vi "Avocent_controller.vi"() -> ()   [LabVIEW 2013]
doc: "Example of using standard HTTP protocol for recieving a web site (the HTML source)\n\n\nThis example uses the GET command. For general information about the HTTP protocol and other commands go to\nhttp://www.w3.org/Protocols\n\n\nBjornar Svingen\nbjornar.svingen@sintef.no bjornar.svingen@ktv.no"
uses:
  <vilib>/Utility/config.llb/Read Key (String).vi
  <vilib>/Utility/config.llb/NI_LVConfig.lvlib
panel:
  in  "Set to all on/off av2":bool
  in  "Set to all on/off av1":bool
  in  "toggle av2":bool
  in  "toggle av1":bool
  out "Avocent Labels Av2":string[](array[string])
  out "Avocent Labels Av1":string[](array[string])
  in  "Set to current values 2":bool
  in  "Set to current values":bool
  in  "Get status 2":bool
  in  "send command 2":bool
  out "Power indicator 2":bool[](array[boolean])=[FALSE, FALSE, FALSE, FALSE, FALSE, FALSE, FALSE, FALSE, FALSE, FALSE, FALSE, FALSE, FALSE, TRUE, TRUE, TRUE, FALSE, FALSE, FALSE, FALSE, FALSE, FALSE, FALSE, FALSE, FALSE, FALSE, FALSE, FALSE, FALSE, FALSE, FALSE, FALSE] caption="Power indicator"
  in  "Set switches 2":bool[](array[boolean])=[FALSE, FALSE, FALSE, FALSE, FALSE, FALSE, FALSE, FALSE, FALSE, FALSE, FALSE, FALSE, FALSE, TRUE, TRUE, TRUE] caption="Set Switches"
  in  "Avocent 2 IP":string="192.168.15.5"
  in  "Set switches":bool[](array[boolean])=[FALSE, TRUE, TRUE, FALSE, TRUE, TRUE, TRUE, TRUE, TRUE, TRUE, TRUE, FALSE, TRUE, TRUE, TRUE, FALSE] caption="Set Switches"
  out "Power indicator":bool[](array[boolean])=[FALSE, TRUE, TRUE, FALSE, TRUE, TRUE, TRUE, TRUE, TRUE, TRUE, TRUE, FALSE, TRUE, TRUE, TRUE, FALSE, FALSE, FALSE, FALSE, FALSE, FALSE, FALSE, FALSE, FALSE, FALSE, FALSE, FALSE, FALSE, FALSE, FALSE, FALSE, FALSE]
  in  "Get status":bool
  in  "send command":bool
  in  "Exit":bool
  in  "Avocent 1 IP":string="192.168.14.88"
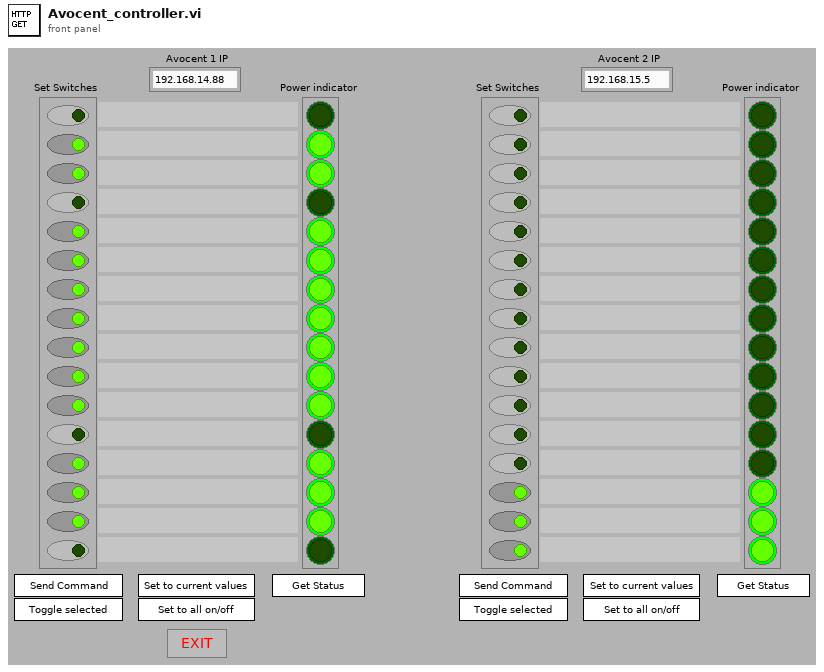
[diagram p1: front panel]
types:
  T1 = enum32{"invalid app kind", "Development System", "Run Time System", "Student Edition", "Embedded LabVIEW", "Evaluation", "Custom"}
  T2 = enum32{"Invalid", "Standard", "Closed", "Hidden", "Minimized", "Maximized"}
  T3 = cluster{"Core":cluster{"Current VI Reference":refnum<vi>, "Close Panel on Exit?":bool}, "HTTP Command":string, "Set Switch Status":bool[], "Power Status":string, "Toggle On/Off":bool, "Set all On/Off":bool}
  T4 = cluster{"Current VI Reference":refnum<vi>, "Close Panel on Exit?":bool}
  T5 = typedef "NI_LVConfig.lvlib/Config Data RefNum.ctl" = refnum<k1>
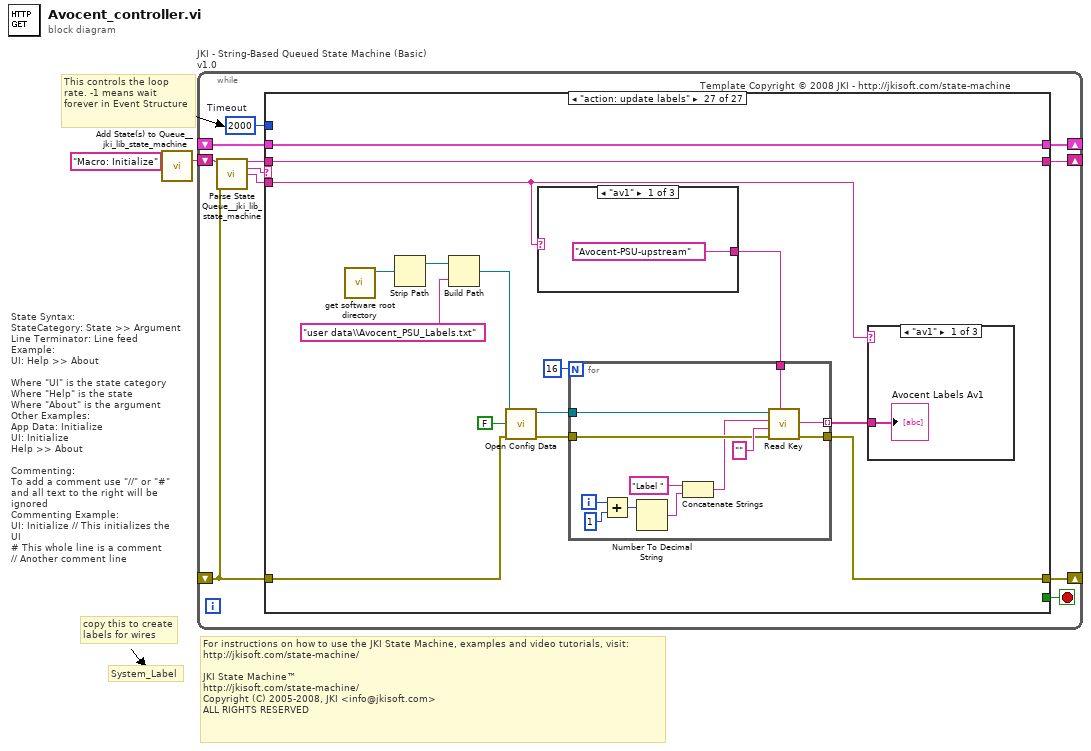
[diagram p0: block diagram]
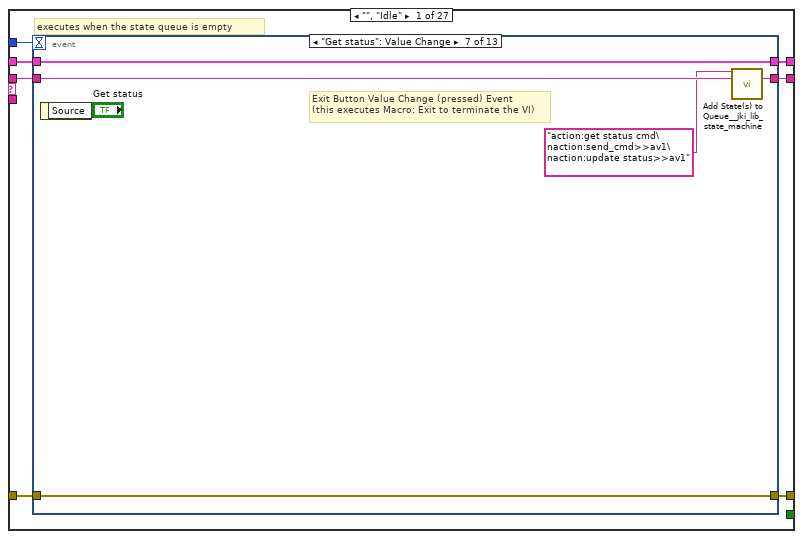
[diagram p2: hidden frame]
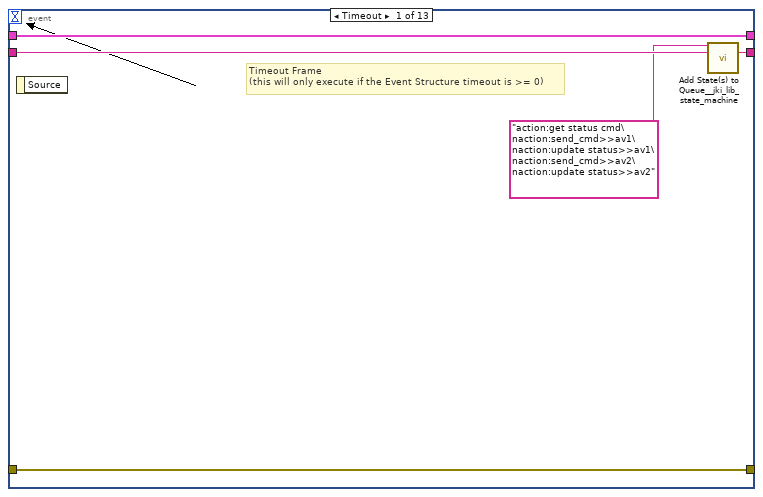
[diagram p3: hidden frame]
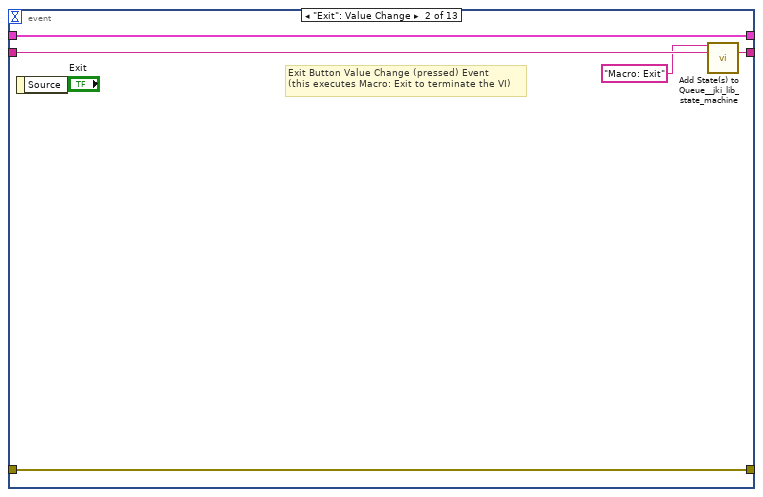
[diagram p4: hidden frame]
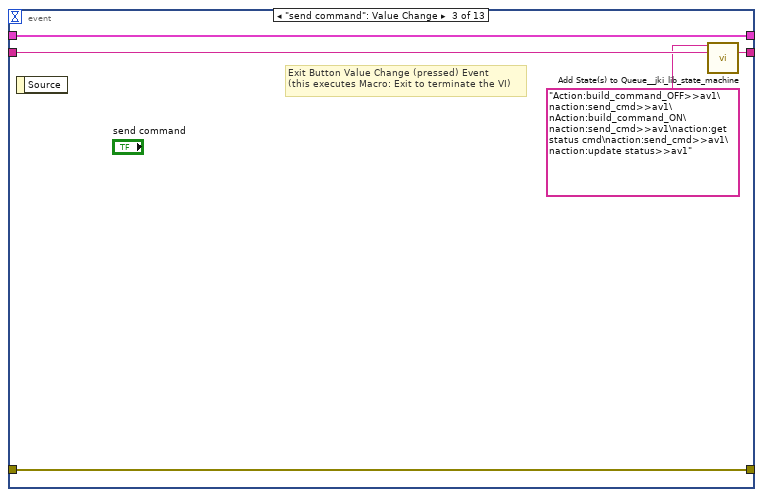
[diagram p5: hidden frame]
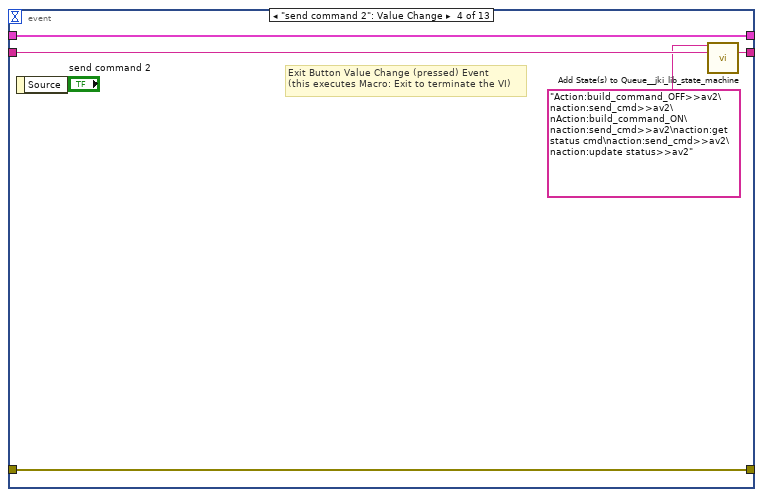
[diagram p6: hidden frame]
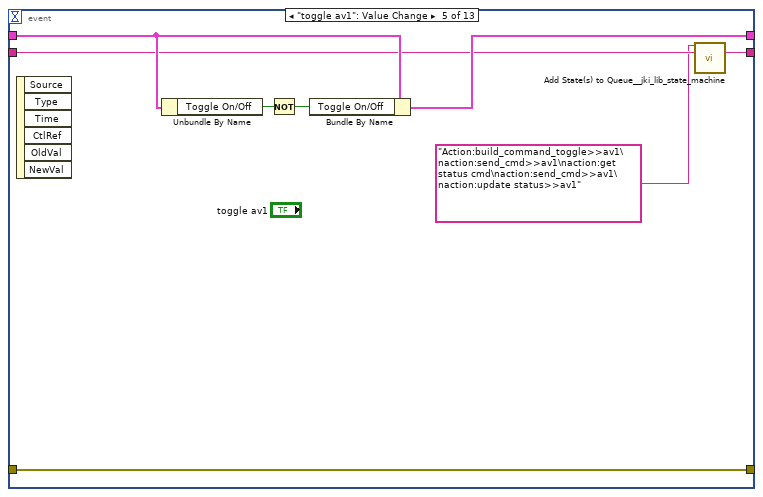
[diagram p7: hidden frame]
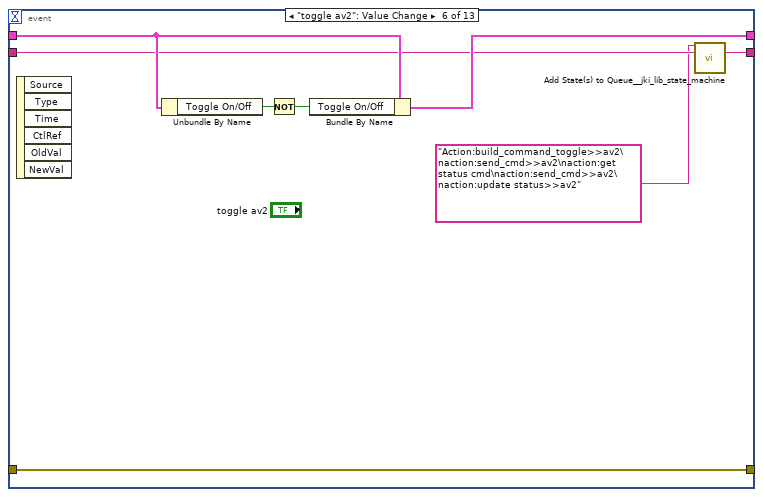
[diagram p8: hidden frame]
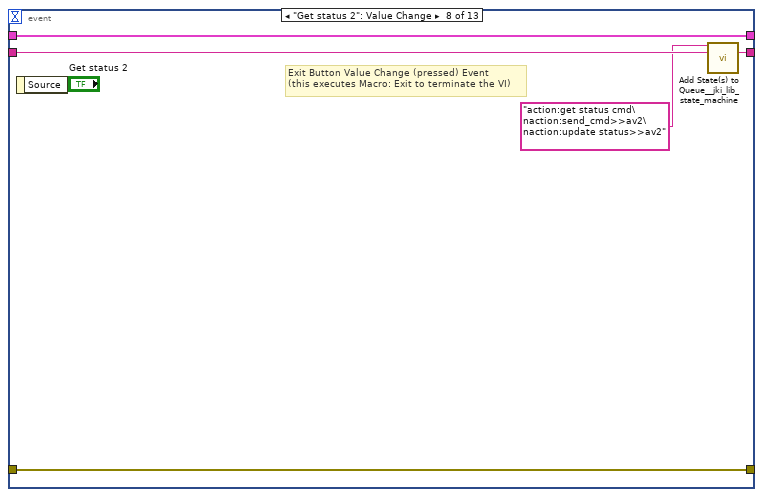
[diagram p9: hidden frame]
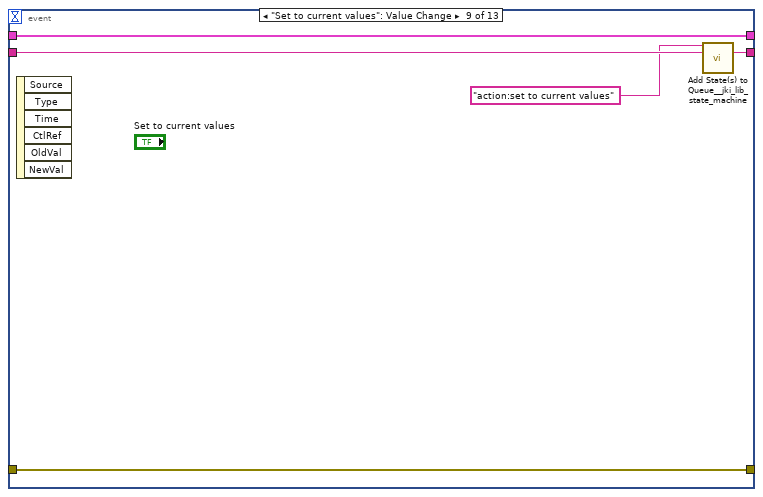
[diagram p10: hidden frame]
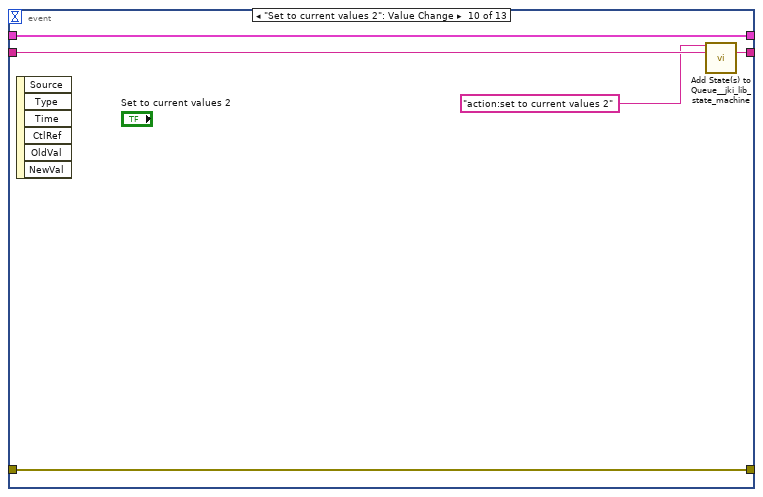
[diagram p11: hidden frame]
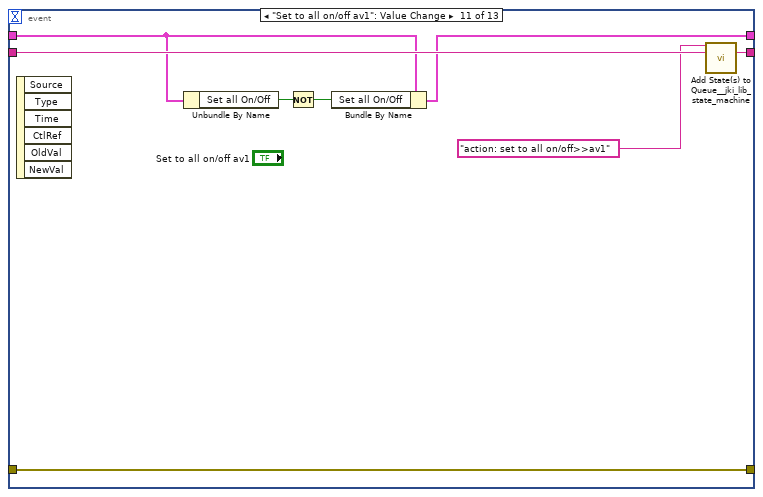
[diagram p12: hidden frame]
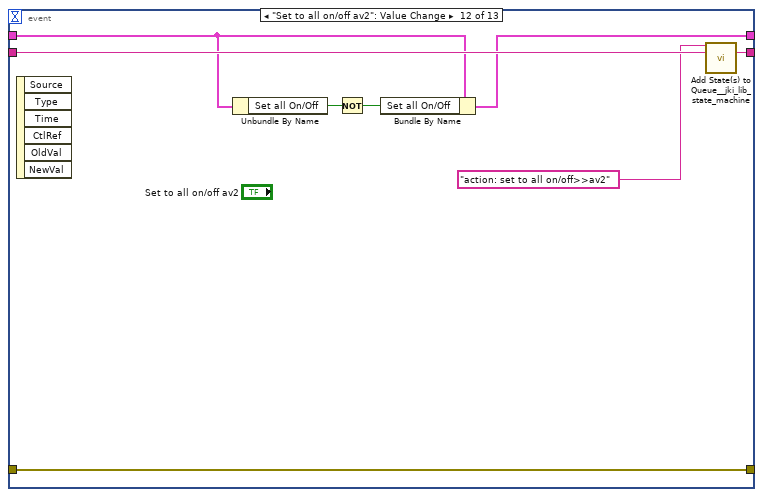
[diagram p13: hidden frame]
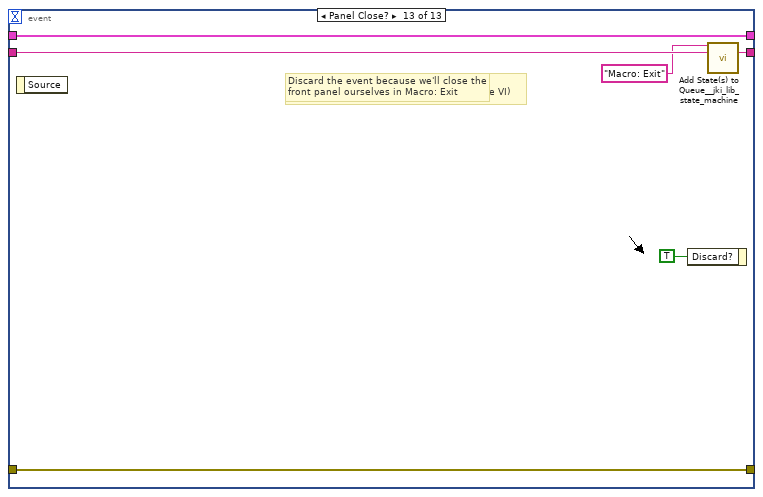
[diagram p14: hidden frame]
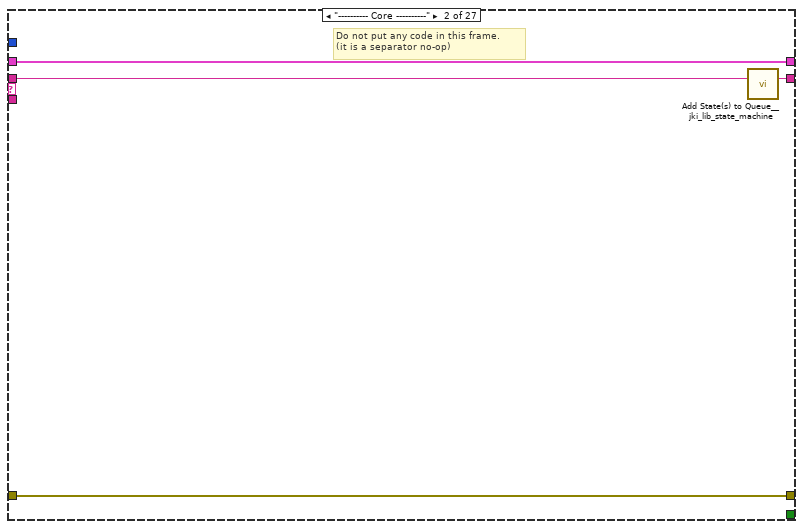
[diagram p15: hidden frame]
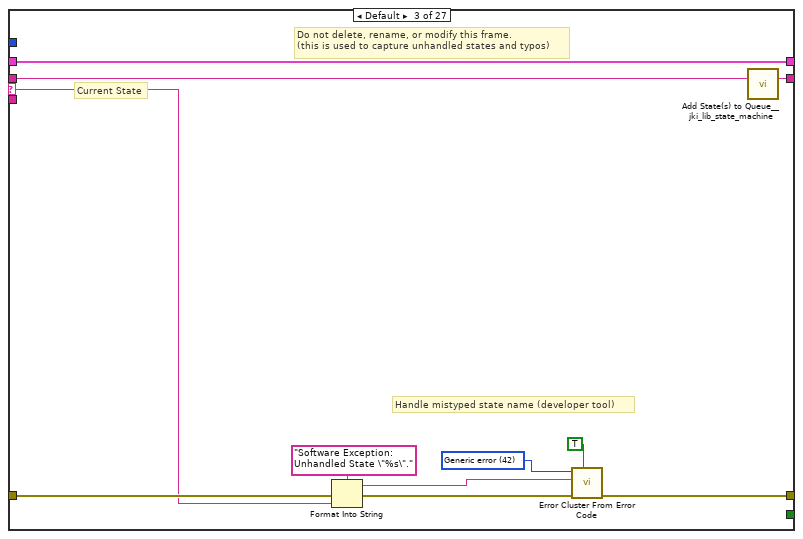
[diagram p16: hidden frame]
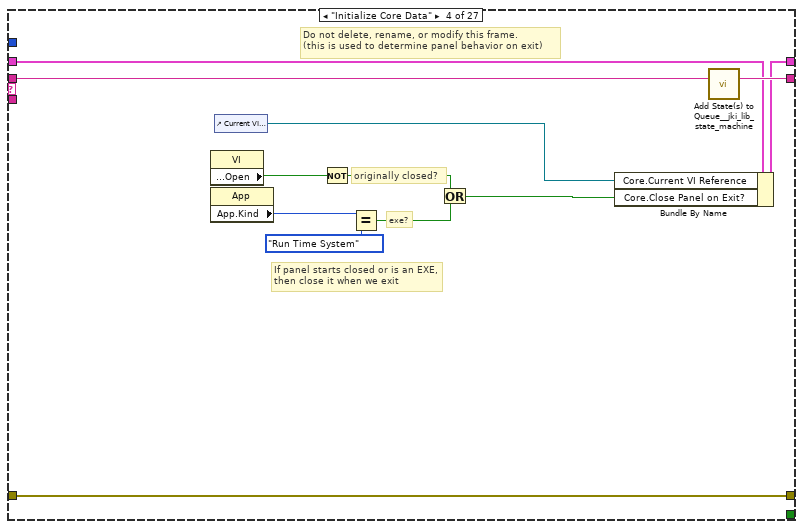
[diagram p17: hidden frame]
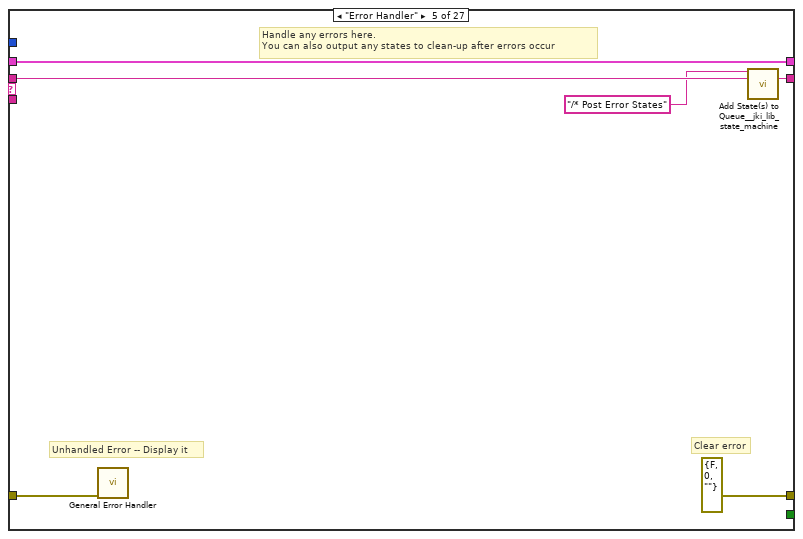
[diagram p18: hidden frame]
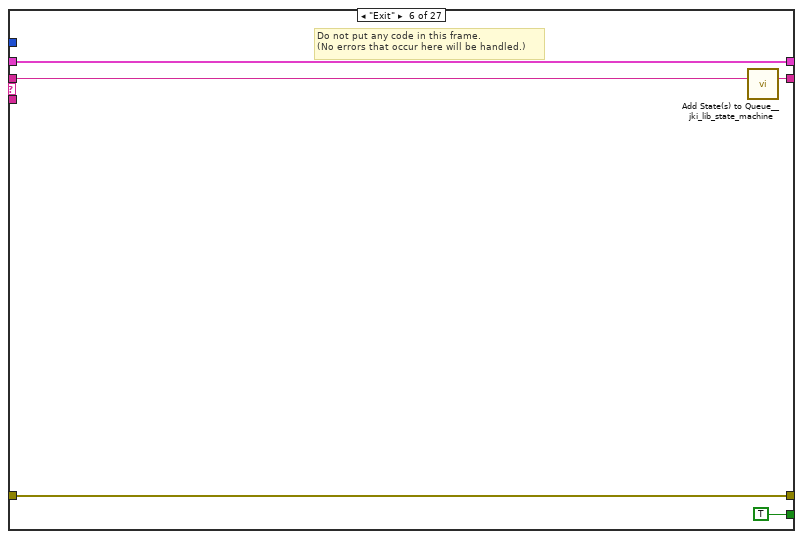
[diagram p19: hidden frame]
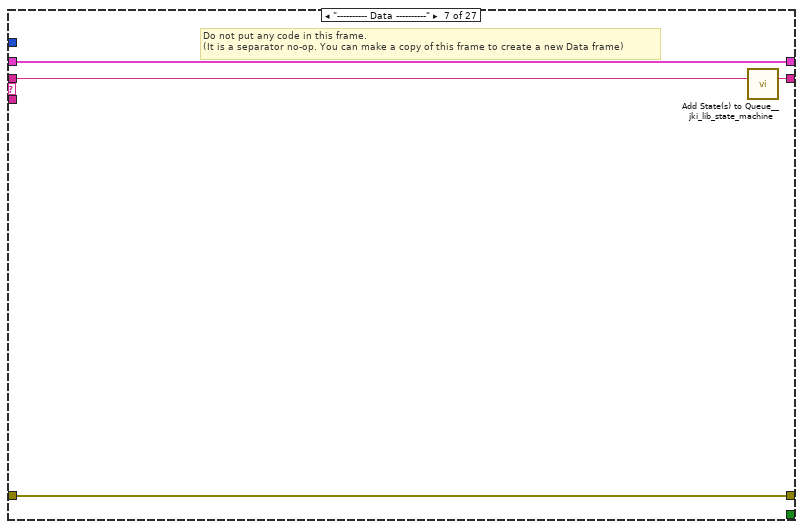
[diagram p20: hidden frame]
diagram:
  # "For instructions on how to use the JKI State Machine, examples and video tutorials, visit:\nhttp://jkisoft.com/state-machine/\n\nJKI State Machine™\nhttp://jkisoft.com/state-machine/\nCopyright (C) 2005-2008, JKI <info@jkisoft.com>\nALL RIGHTS RESERVED"
  # "State Syntax:\nStateCategory: State >> Argument\nLine Terminator: Line feed\nExample:\nUI: Help >> About\n\nWhere \"UI\" is the state category\nWhere \"Help\" is the state\nWhere \"About\" is the argument\nOther Examples:\nApp Data: Initialize\nUI: Initialize\nHelp >> About\n\nCommenting:\nTo add a comment use \"//\" or \"#\" and all text to the right will be ignored\nCommenting Example:\nUI: Initialize // This initializes the UI\n# This whole line is a comment\n// Another comment line"
  # "copy this to create labels for wires"
  # "This controls the loop rate. -1 means wait forever in Event Structure"
  # "System_Label"
  n1 = call <vilib>:"Add State(s) to Queue__jki_lib_state_machine.vi"("State(s) in (\"\")"="Macro: Initialize") -> ("States Out"=w2:string)  [unwired: 14 in]
  n2 = while "JKI - String-Based Queued State Machine (Basic) v1.0" {
    shift-right: [w6] -> _
    shift-left: _ -> [w5]
    shift-right: [w9] -> _
    shift-left: _ -> [w3]
    shift-right: [w8] -> _
    shift-left: w2 -> [w10]
    stop <- w7 stop-if-true
    w4 = 2000  # Timeout
    # "Template Copyright © 2008 JKI - http://jkisoft.com/state-machine"
    n3 = call <vilib>:"Parse State Queue__jki_lib_state_machine.vi"("State Queue"=w10, "Error In (no error)"=w3) -> ("Remaining States"=w12:string, "Current State"=w13:string, "Arguments"=w11:string)  [unwired: 11 in]
    n4 = case shown="\"action: update labels\"" w13 {
      selector: w13 -> [_ _ w103 _ _ _ _ _ _ _ _ _ _ _ _ _ _ _ _ _ _ _ _ _ _ _ _]
      tunnel: w12 -> [w20 w102 w107 w125 w131 w136 w140 w150 w156 w160 w164 w170 w181 w207 w212 w222 w226 w228 w252 w272 w277 w297 w316 w323 w330 w336 w364]
      tunnel: w11 -> [_ _ _ _ _ _ _ _ _ _ _ w165 w175 _ _ _ _ w231 w253 _ w279 w300 _ _ _ w337 w351]
      tunnel: w5 -> [w18 w99 w105 w116 w128 w134 w137 _ w151 w157 w162 w168 w177 w204 w209 w219 w223 w233 w256 w268 w278 w301 w313 w321 w328 w332 w365]
      tunnel: [w17 w100 w109 w122 errorcluster {"status"=FALSE, "code"=0, "source"=""} ("error out") w133 w138 w147 w152 w158 w161 w166 w178 w205 w210 w220 w224 w236 w250 w270 w280 w298 w314 w318 w326 w338 w355] -> w9
      tunnel: w3 -> [w16 w100 w108 w122 w127 w133 w138 w147 w153 w158 w161 w167 w179 w205 w210 w220 w224 w230 w251 w270 w281 w299 w314 w319 w327 w339 w356]
      tunnel: [w19 w101 w106 w124 w130 w135 w139 w149 w155 w159 w163 w169 w180 w206 w211 w221 w225 w238 w257 w271 w283 w302 w315 w322 w329 w340 w364] -> w8
      tunnel: [_ _ _ _ _ TRUE _ _ _ _ _ _ _ _ _ _ _ _ _ _ _ _ _ _ _ _ _] -> w7
      tunnel: [w15 w99 w105 w123 w128 w134 w137 w148 w151 w157 w162 w168 w177 w204 w209 w219 w223 w232 w254 w269 w282 w301 w312 w321 w328 w332 w365] -> w6
      tunnel: w4 -> [w14 _ _ _ _ _ _ _ _ _ _ _ _ _ _ _ _ _ _ _ _ _ _ _ _ _ _]
      frame "", "Idle" {
        # "executes when the state queue is empty"
        n5 = event shown="[6] \"Get status\": Value Change" {
          selector: _ -> [_ _ _ _ _ _ _ _ _ _ _ _ _]
          dyn-events: _ -> [_ _ _ _ _ _ _ _ _ _ _ _ _]
          timeout: w14 -> [_ _ _ _ _ _ _ _ _ _ _ _ _]
          tunnel: w20 -> [w25 w30 w35 w40 w43 w51 w61 w66 w68 w73 w82 w90 w98]
          tunnel: [w24 w29 w34 w39 w42 w50 w60 w65 w69 w74 w83 w91 w97] -> w19
          tunnel: w18 -> [w22 w27 w32 w37 w46 w54 w58 w63 w71 w76 w78 w86 w95]
          tunnel: [w23 w28 w33 w38 w48 w56 w59 w64 w70 w75 w84 w92 w96] -> w17
          tunnel: w16 -> [w23 w28 w33 w38 w48 w56 w59 w64 w70 w75 w84 w92 w96]
          tunnel: [w22 w27 w32 w37 w47 w55 w58 w63 w71 w76 w77 w85 w95] -> w15
          event Timeout {
            # "Timeout Frame\n(this will only execute if the Event Structure timeout is >= 0)"
            n6 = event-data() -> ()  [unwired: 1 in, 1 out]
            n7 = call <vilib>:"Add State(s) to Queue__jki_lib_state_machine.vi"("State(s) in Front (\"\")"="action:get status cmd\naction:send_cmd>>av1\naction:update status>>av1\naction:send_cmd>>av2\naction:update status>>av2", "State(s) in (\"\")"=w25) -> ("States Out"=w24:string)  [unwired: 13 in]
          }
          event "Exit": Value Change {
            # "Exit Button Value Change (pressed) Event\n(this executes Macro: Exit to terminate the VI)"
            n8 = event-data() -> ()  [unwired: 1 in, 1 out]
            n9 = call <vilib>:"Add State(s) to Queue__jki_lib_state_machine.vi"("State(s) in Front (\"\")"="Macro: Exit", "State(s) in (\"\")"=w30) -> ("States Out"=w29:string)  [unwired: 13 in]
          }
          event "send command": Value Change {
            # "Exit Button Value Change (pressed) Event\n(this executes Macro: Exit to terminate the VI)"
            n10 = event-data() -> ()  [unwired: 1 in, 1 out]
            n11 = call <vilib>:"Add State(s) to Queue__jki_lib_state_machine.vi"("State(s) in Front (\"\")"="Action:build_command_OFF>>av1\naction:send_cmd>>av1\nAction:build_command_ON\naction:send_cmd>>av1\naction:get status cmd\naction:send_cmd>>av1\naction:update status>>av1", "State(s) in (\"\")"=w35) -> ("States Out"=w34:string)  [unwired: 13 in]
          }
          event "send command 2": Value Change {
            # "Exit Button Value Change (pressed) Event\n(this executes Macro: Exit to terminate the VI)"
            n12 = event-data() -> ()  [unwired: 1 in, 1 out]
            n13 = call <vilib>:"Add State(s) to Queue__jki_lib_state_machine.vi"("State(s) in Front (\"\")"="Action:build_command_OFF>>av2\naction:send_cmd>>av2\nAction:build_command_ON\naction:send_cmd>>av2\naction:get status cmd\naction:send_cmd>>av2\naction:update status>>av2", "State(s) in (\"\")"=w40) -> ("States Out"=w39:string)  [unwired: 13 in]
          }
          event "toggle av1": Value Change {
            n14 = event-data() -> ()  [unwired: 1 in, 6 out]
            n15 = Unbundle By Name(w46) -> ("Toggle On/Off"=w45:bool)
            n16 = Not(x=w45) -> (.not. x?=w44:bool)
            n17 = Bundle By Name(cluster=w46, "Toggle On/Off"=w44) -> (w47:T3)
            n18 = call <vilib>:"Add State(s) to Queue__jki_lib_state_machine.vi"("State(s) in Front (\"\")"="Action:build_command_toggle>>av1\naction:send_cmd>>av1\naction:get status cmd\naction:send_cmd>>av1\naction:update status>>av1", "State(s) in (\"\")"=w43) -> ("States Out"=w42:string)  [unwired: 13 in]
          }
          event "toggle av2": Value Change {
            n19 = event-data() -> ()  [unwired: 1 in, 6 out]
            n20 = Unbundle By Name(w54) -> ("Toggle On/Off"=w53:bool)
            n21 = Not(x=w53) -> (.not. x?=w52:bool)
            n22 = Bundle By Name(cluster=w54, "Toggle On/Off"=w52) -> (w55:T3)
            n23 = call <vilib>:"Add State(s) to Queue__jki_lib_state_machine.vi"("State(s) in Front (\"\")"="Action:build_command_toggle>>av2\naction:send_cmd>>av2\naction:get status cmd\naction:send_cmd>>av2\naction:update status>>av2", "State(s) in (\"\")"=w51) -> ("States Out"=w50:string)  [unwired: 13 in]
          }
          event "Get status": Value Change {
            # "Exit Button Value Change (pressed) Event\n(this executes Macro: Exit to terminate the VI)"
            n24 = event-data() -> ()  [unwired: 1 in, 1 out]
            n25 = call <vilib>:"Add State(s) to Queue__jki_lib_state_machine.vi"("State(s) in Front (\"\")"="action:get status cmd\naction:send_cmd>>av1\naction:update status>>av1", "State(s) in (\"\")"=w61) -> ("States Out"=w60:string)  [unwired: 13 in]
          }
          event "Get status 2": Value Change {
            # "Exit Button Value Change (pressed) Event\n(this executes Macro: Exit to terminate the VI)"
            n26 = event-data() -> ()  [unwired: 1 in, 1 out]
            n27 = call <vilib>:"Add State(s) to Queue__jki_lib_state_machine.vi"("State(s) in Front (\"\")"="action:get status cmd\naction:send_cmd>>av2\naction:update status>>av2", "State(s) in (\"\")"=w66) -> ("States Out"=w65:string)  [unwired: 13 in]
          }
          event "Set to current values": Value Change {
            n28 = event-data() -> ()  [unwired: 1 in, 6 out]
            n29 = call <vilib>:"Add State(s) to Queue__jki_lib_state_machine.vi"("State(s) in Front (\"\")"="action:set to current values" ("State(s) in Front (\"\")"), "State(s) in (\"\")"=w68) -> ("States Out"=w69:string)  [unwired: 13 in]
          }
          event "Set to current values 2": Value Change {
            n30 = event-data() -> ()  [unwired: 1 in, 6 out]
            n31 = call <vilib>:"Add State(s) to Queue__jki_lib_state_machine.vi"("State(s) in Front (\"\")"="action:set to current values 2" ("State(s) in Front (\"\")"), "State(s) in (\"\")"=w73) -> ("States Out"=w74:string)  [unwired: 13 in]
          }
          event "Set to all on/off av1": Value Change {
            n32 = event-data() -> ()  [unwired: 1 in, 6 out]
            n33 = Unbundle By Name(w78) -> ("Set all On/Off"=w80:bool)
            n34 = Not(x=w80) -> (.not. x?=w79:bool)
            n35 = Bundle By Name(cluster=w78, "Set all On/Off"=w79) -> (w77:T3)
            n36 = call <vilib>:"Add State(s) to Queue__jki_lib_state_machine.vi"("State(s) in Front (\"\")"="action: set to all on/off>>av1" ("State(s) in Front (\"\")"), "State(s) in (\"\")"=w82) -> ("States Out"=w83:string)  [unwired: 13 in]
          }
          event "Set to all on/off av2": Value Change {
            n37 = event-data() -> ()  [unwired: 1 in, 6 out]
            n38 = Unbundle By Name(w86) -> ("Set all On/Off"=w88:bool)
            n39 = Not(x=w88) -> (.not. x?=w87:bool)
            n40 = Bundle By Name(cluster=w86, "Set all On/Off"=w87) -> (w85:T3)
            n41 = call <vilib>:"Add State(s) to Queue__jki_lib_state_machine.vi"("State(s) in Front (\"\")"="action: set to all on/off>>av2" ("State(s) in Front (\"\")"), "State(s) in (\"\")"=w90) -> ("States Out"=w91:string)  [unwired: 13 in]
          }
          event Panel Close? {
            # "Discard the event because we'll close the front panel ourselves in Macro: Exit"
            # "Close Panel button (pressed) Event\n(this executes Macro: Exit to terminate the VI)"
            n42 = event-data() -> ()  [unwired: 1 in, 1 out]
            n43 = event-data("Discard?"=TRUE) -> ()  [unwired: 1 in, 1 out]
            n44 = call <vilib>:"Add State(s) to Queue__jki_lib_state_machine.vi"("State(s) in Front (\"\")"="Macro: Exit", "State(s) in (\"\")"=w98) -> ("States Out"=w97:string)  [unwired: 13 in]
          }
        }
      }
      frame "---------- Core ----------" {
        # "Do not put any code in this frame.\n(it is a separator no-op)"
        n45 = call <vilib>:"Add State(s) to Queue__jki_lib_state_machine.vi"("State(s) in (\"\")"=w102) -> ("States Out"=w101:string)  [unwired: 14 in]
      }
      frame Default {
        w112 = 42 items=["No error", "Argument error", "Memory is full", "Out of zone", "End of file", "File already open", "Generic file I/O error", "File not found", "File permission error", "Disk is full", "Duplicate path", "Too many files open", "System feature not enabled", "Resource file not found", "Cannot add resource", "Resource not found", "Image not found", "Image memory error", "Pen does not exist", "Config type invalid", "Config token not found", "Config parse error", "Config memory error", "Bad external code format", "Bad external code offset", "External code not present", "Null window", "Destroy window error", "Null menu", "Print aborted", "Bad print record", "Print driver error", "Windows error during printing", "Memory error during printing", "Print dialog error", "Generic print error", "Invalid device refnum", "Device not found", "Device parameter error", "Device unit error", "Cannot open device", "Device call aborted", "Generic error", "Cancelled by user", "Object ID too low", "Object ID too high", "Object not in heap", "Unknown heap", "Unknown object (invalid DefProc)", "Unknown object (DefProc not in table)", "Message out of range", "Invalid (null) method", "Unknown message", "Manager call not supported", "Bad address", "Network operation in progress", "Network operation timed out", "Connection is busy", "Network attribute not supported", "Network error", "Address in use", "System out of memory", "Connection aborted", "Connection refused", "Not connected", "Already connected", "Connection closed", "Initialization error (interapplication manager)", "Bad occurrence", "Wait on unbound occurrence handler", "Occurrence queue overflow", "Datalog type conflict", "Unused", "Unrecognized type (interapplication manager)", "Memory corrupt", "Failed to make temporary DLL", "Old CIN version", "Drag socket not found", "Failed to load drop-object", "Failed to register OLE object", "Failed to release OLE object", "Format specifier type mismatch", "Unknown format specifier", "Too few format specifiers", "Too many format specifiers", "Scan failed", "Newer CIN version", "Error converting to variant", "Runtime menu error", "Password tampered", "Variant attribute not found", "Incompatible variant data type", "Event data is not available", "Event Store is not present", "Occurrence is not found", "Event Queue is not created", "Event info is not available", "Refnum passed is NULL", "Error retrieving Class GUID", "Error retrieving CoClass GUID", "Error retrieving TypeLib GUID.", "Bad built application magic bytes.", "Specific driver is different from the specific driver associated with the Logical Name.", "There is no session opened to the class driver.", "Max Error", "MAX - Error with config objects", "MAX - Error loading configuration", "MAX - Group not supported"]
        # "Current State"
        # "Do not delete, rename, or modify this frame.\n(this is used to capture unhandled states and typos)"
        # "Handle mistyped state name (developer tool)"
        n46 = Format Into String(format string="Software Exception: Unhandled State \"%s\"." ("message"), error in=w108, w103) -> (resulting string=w111:string, error out=w110:errorcluster)  [unwired: 1 in]
        n47 = call <vilib>:"Error Cluster From Error Code.vi"("show call chain? (False)"=TRUE, "error in (no error)"=w110, "error message (\"\")"=w111, "error code (0)"=w112) -> ("error out"=w109:errorcluster)  [unwired: 5 in]
        n48 = call <vilib>:"Add State(s) to Queue__jki_lib_state_machine.vi"("State(s) in (\"\")"=w107) -> ("States Out"=w106:string)  [unwired: 14 in]
      }
      frame "Initialize Core Data" {
        # "Do not delete, rename, or modify this frame.\n(this is used to determine panel behavior on exit)"
        # "originally closed?"
        # "exe?"
        # "If panel starts closed or is an EXE, then close it when we exit"
        n49 = property class="VI"() -> ("Front Panel.Open"=w121:bool)  [unwired: 2 in, 2 out]
        n50 = property class="App"() -> ("App.Kind"=w120:T1)  [unwired: 2 in, 2 out]
        n51 = control-ref of="Current VI Reference"() -> (w114:refnum<vi>)
        n52 = Not(x=w121) -> (.not. x?=w118:bool)
        n53 = Equal?(x=w120, y=T1."Run Time System" ("Application:Kind")) -> (x = y?=w117:bool)
        n54 = Or(x=w118, y=w117) -> (x .or. y?=w115:bool)
        n55 = Bundle By Name(cluster=w116, "Core.Current VI Reference"=w114, "Core.Close Panel on Exit?"=w115) -> (w123:T3)
        n56 = call <vilib>:"Add State(s) to Queue__jki_lib_state_machine.vi"("State(s) in (\"\")"=w125) -> ("States Out"=w124:string)  [unwired: 14 in]
      }
      frame "Error Handler" {
        # "Unhandled Error -- Display it"
        # "Handle any errors here.\nYou can also output any states to clean-up after errors occur"
        # "Clear error"
        n57 = call <vilib>:"General Error Handler.vi"("error in (no error)"=w127) -> ()  [unwired: 10 in, 5 out]
        n58 = call <vilib>:"Add State(s) to Queue__jki_lib_state_machine.vi"("State(s) in Front (\"\")"="/* Post Error States", "State(s) in (\"\")"=w131) -> ("States Out"=w130:string)  [unwired: 13 in]
      }
      frame "Exit" {
        # "Do not put any code in this frame.\n(No errors that occur here will be handled.)"
        n59 = call <vilib>:"Add State(s) to Queue__jki_lib_state_machine.vi"("State(s) in (\"\")"=w136) -> ("States Out"=w135:string)  [unwired: 14 in]
      }
      frame "---------- Data ----------" {
        # "Do not put any code in this frame.\n(It is a separator no-op. You can make a copy of this frame to create a new Data frame)"
        n60 = call <vilib>:"Add State(s) to Queue__jki_lib_state_machine.vi"("State(s) in (\"\")"=w140) -> ("States Out"=w139:string)  [unwired: 14 in]
      }
      frame "Data: Initialize" {
        w141 = TRUE  # Set all On/Off
        w142 = bool[] [FALSE, FALSE, FALSE, FALSE, FALSE, FALSE, FALSE, FALSE, FALSE, TRUE, FALSE, FALSE, FALSE, FALSE, FALSE, FALSE, FALSE, FALSE, FALSE, FALSE, FALSE, FALSE, FALSE, FALSE, FALSE, FALSE, FALSE, FALSE, FALSE, FALSE, FALSE, FALSE]  # Set Switch Status
        w143 = TRUE  # Toggle On/Off
        w144 = ""  # Power Status
        w145 = ""  # HTTP Command
        w146 = T4 {"Current VI Reference"=refnum, "Close Panel on Exit?"=FALSE}  # Core
        # "do not delete - used by framework"
        # "Add new data here."
        # "Data names and types of shift register data are defined by this bundle."
        # "Initialize the shift-register data, here.\n(data names are defined by what you wire into the bundle function)"
        n61 = Bundle("Core"=w146, "HTTP Command"=w145, "Set Switch Status"=w142, "Power Status"=w144, "Toggle On/Off"=w143, "Set all On/Off"=w141) -> (w148:T3)  [unwired: 1 in]
        n62 = call <vilib>:"Add State(s) to Queue__jki_lib_state_machine.vi"("State(s) in (\"\")"=w150) -> ("States Out"=w149:string)  [unwired: 14 in]
      }
      frame "Data: Cleanup" {
        # "Cleanup any data and references, here.\n(this is called automatically, by the Macro: Exit)"
        n63 = Unbundle By Name(w151) -> ("Core.Current VI Reference"=w154:refnum<vi>)
        n64 = Close Reference(reference=w154, error in (no error)=w153) -> (error out=w152:errorcluster)
        n65 = call <vilib>:"Add State(s) to Queue__jki_lib_state_machine.vi"("State(s) in (\"\")"=w156) -> ("States Out"=w155:string)  [unwired: 14 in]
      }
      frame "---------- UI ----------" {
        # "Do not put any code in this frame.\n(It is a separator no-op. You can make a copy of this frame to create a new UI frame)"
        n66 = call <vilib>:"Add State(s) to Queue__jki_lib_state_machine.vi"("State(s) in (\"\")"=w160) -> ("States Out"=w159:string)  [unwired: 14 in]
      }
      frame "UI: Initialize" {
        # "Initialize the User Interface, here.\n(this is called automatically, by the Macro: Init)"
        n67 = call <vilib>:"Add State(s) to Queue__jki_lib_state_machine.vi"("State(s) in (\"\")"=w164) -> ("States Out"=w163:string)  [unwired: 14 in]
      }
      frame "UI: Cursor Set" {
        # "Argument"
        # "Set and Unset Cursor Busy.\n(Usage: \"UI: Cursor Set >> Busy|Idle\")"
        n68 = case shown="\"Idle\", Default" w165 {
          tunnel: w167 -> [w172 w174]
          tunnel: [w171 w173] -> w166
          frame "Idle", Default {
            n69 = call <vilib>:"Unset Busy.vi"("error in (no error)"=w172) -> ("error out"=w171:errorcluster)  [unwired: 10 in]
          }
          frame "Busy" {
            n70 = call <vilib>:"Set Busy.vi"("error in (no error)"=w174) -> ("error out"=w173:errorcluster)  [unwired: 9 in, 1 out]
          }
        }
        n71 = call <vilib>:"Add State(s) to Queue__jki_lib_state_machine.vi"("State(s) in (\"\")"=w170) -> ("States Out"=w169:string)  [unwired: 14 in]
      }
      frame "UI: Front Panel State" {
        # "Argument"
        # "Set Front Panel Open or Closed\n(Usage: \"UI: Front Panel State >> Open|Close\")"
        n72 = Unbundle By Name(w177) -> ("Core.Current VI Reference"=w176:refnum<vi>)
        n73 = case shown="\"Open\", Default" w175 {
          tunnel: w179 -> [w185 w198]
          tunnel: [w187 w199] -> w178
          tunnel: w176 -> [w186 w196]
          frame "Open", Default {
            n74 = property class="VI"(reference=w186, error in=w185) -> (reference out=w183:refnum<vi>, error out=w184:errorcluster, "Front Panel.Open"=w182:bool)
            n75 = case shown="False" w182 {
              tunnel: [w190 w193] -> w187
              tunnel: w184 -> [w189 w193]
              tunnel: w183 -> [w188 _]
              frame False {
                n76 = invoke class="VI" method="FP.Open"(reference=w188, error in=w189, "Activate"=TRUE, "State"=T2."Standard") -> (error out=w190:errorcluster)  [unwired: 1 in, 4 out]
              }
              frame True {
              }
            }
          }
          frame "Close" {
            n77 = property class="VI"(reference=w196, error in=w198) -> (reference out=w195:refnum<vi>, error out=w197:errorcluster, "Front Panel.Open"=w194:bool)
            n78 = case shown="True" w194 {
              tunnel: [w200 w203] -> w199
              tunnel: w197 -> [w200 w202]
              tunnel: w195 -> [_ w201]
              frame False {
              }
              frame True {
                n79 = invoke class="VI" method="FP.Close"(reference=w201, error in=w202) -> (error out=w203:errorcluster)  [unwired: 1 in, 2 out]
              }
            }
          }
        }
        n80 = call <vilib>:"Add State(s) to Queue__jki_lib_state_machine.vi"("State(s) in (\"\")"=w181) -> ("States Out"=w180:string)  [unwired: 14 in]
      }
      frame "---------- Macro ----------" {
        # "Do not put any code in this frame.\n(It is a separator no-op. You can make a copy of this frame to create a new Macro frame)"
        n81 = call <vilib>:"Add State(s) to Queue__jki_lib_state_machine.vi"("State(s) in (\"\")"=w207) -> ("States Out"=w206:string)  [unwired: 14 in]
      }
      frame "Macro: Initialize" {
        w208 = "Data: Initialize\nInitialize Core Data\nUI: Initialize\nUI: Front Panel State >> Open\naction: update labels>>av1\naction: update labels>>av2\naction:get status cmd\naction:send_cmd>>av1\naction:update status>>av1\naction:set to current values\naction:send_cmd>>av2\naction:update status>>av2\naction:set to current values 2"  # Data: Initialize Initialize Core Data UI: Initialize UI: Front Panel State >> Open action: update labels>>av1 action: update labels>>av2 action:get status cmd action:send_cmd>>av1 action:update status>>av1 action:set to current values action:send_cmd>>av2 action:update status>>av2 action:set to current values 2
        # "Initialization Macro\n(This is called once, when the VI starts)"
        n82 = call <vilib>:"Add State(s) to Queue__jki_lib_state_machine.vi"("State(s) in Front (\"\")"=w208, "State(s) in (\"\")"=w212) -> ("States Out"=w211:string)  [unwired: 13 in]
      }
      frame "Macro: Exit" {
        # "Exit Macro\n(This is called once, when the VI exits)"
        n83 = Unbundle By Name(w219) -> ("Core.Close Panel on Exit?"=w218:bool)
        n84 = Select(t="UI: Front Panel State >> Close", s=w218, f="") -> (s? t:f=w215:string)
        n85 = call <vilib>:"Add State(s) to Queue__jki_lib_state_machine.vi"("State(s) in (\"\")"=w215, "State(s) at Back (\"\")"="Data: Cleanup\nExit") -> ("States Out"=w213:string)  [unwired: 13 in]
        n86 = call <vilib>:"Add State(s) to Queue__jki_lib_state_machine.vi"("State(s) in Front (\"\")"=w213, "State(s) in (\"\")"=w222) -> ("States Out"=w221:string)  [unwired: 13 in]
      }
      frame "---------- New Category ----------" {
        # "Template Separator\n(You can make a copy of, or modify, this frame)"
        n87 = call <vilib>:"Add State(s) to Queue__jki_lib_state_machine.vi"("State(s) in (\"\")"=w226) -> ("States Out"=w225:string)  [unwired: 14 in]
      }
      frame "action:send_cmd" {
        # "Your code here.\n(You can make a copy of, or modify, this frame)"
        n88 = case shown="\"av1\"" w231 {
          tunnel: ["Avocent 2 IP" _ "Avocent 1 IP"] -> w237
          tunnel: [w240 errorcluster {"status"=TRUE, "code"=0, "source"="Error:\nno avocent selected"} ("error out") w245] -> w229
          tunnel: w230 -> [w240 _ w245]
          tunnel: [w239 "" w244] -> w227
          tunnel: w228 -> [w239 _ w244]
          frame "av2" {
          }
          frame Default {
          }
          frame "av1" {
          }
        }
        n89 = Unbundle By Name(w233) -> ("HTTP Command"=w235:string)
        n90 = call "Avocent_send_cmd.vi"("error in"=w229, "Avocent IP (in)"=w237, "HTTP command"=w235) -> ("error out"=w236:errorcluster, "Replay"=w234:string)  [unwired: 6 in, 1 out]
        n91 = Bundle By Name(cluster=w233, "Power Status"=w234) -> (w232:T3)
        n92 = call <vilib>:"Add State(s) to Queue__jki_lib_state_machine.vi"("State(s) in (\"\")"=w227) -> ("States Out"=w238:string)  [unwired: 14 in]
      }
      frame "Action:build_command_OFF" {
        # "Your code here.\n(You can make a copy of, or modify, this frame)"
        n93 = case shown="\"av1\"" w253 {
          tunnel: ["Set switches 2" _ "Set switches"] -> w248
          tunnel: [w258 "" w264] -> w249
          tunnel: w252 -> [w258 _ w264]
          tunnel: w251 -> [w259 _ w263]
          tunnel: [w259 errorcluster {"status"=TRUE, "code"=0, "source"="Error:\nno avocent selected"} ("error out") w263] -> w250
          frame "av2" {
          }
          frame Default {
          }
          frame "av1" {
          }
        }
        n94 = call "Avocent_build_command_OFF.vi"("Set switches"=w248) -> ("HTTP command"=w247:string)  [unwired: 10 in]
        n95 = Bundle By Name(cluster=w256, "Set Switch Status"=w248) -> (w255:T3)
        n96 = Bundle By Name(cluster=w255, "HTTP Command"=w247) -> (w254:T3)
        n97 = call <vilib>:"Add State(s) to Queue__jki_lib_state_machine.vi"("State(s) in (\"\")"=w249) -> ("States Out"=w257:string)  [unwired: 14 in]
      }
      frame "Action:build_command_ON" {
        # "Your code here.\n(You can make a copy of, or modify, this frame)"
        n98 = Unbundle By Name(w268) -> ("Set Switch Status"=w266:bool[])
        n99 = call "Avocent_build_command_ON.vi"("Set switches"=w266) -> ("HTTP command"=w267:string)  [unwired: 10 in]
        n100 = Bundle By Name(cluster=w268, "HTTP Command"=w267) -> (w269:T3)
        n101 = call <vilib>:"Add State(s) to Queue__jki_lib_state_machine.vi"("State(s) in (\"\")"=w272) -> ("States Out"=w271:string)  [unwired: 14 in]
      }
      frame "Action:build_command_toggle" {
        # "Your code here.\n(You can make a copy of, or modify, this frame)"
        n102 = case shown="Default" w279 {
          tunnel: [w287 _ w293] -> w273
          tunnel: w281 -> [w286 _ w292]
          tunnel: [w285 errorcluster {"status"=TRUE, "code"=0, "source"="Error:\nno avocent selected"} ("error out") w291] -> w280
          tunnel: w277 -> [w284 _ w290]
          tunnel: [w284 "" w290] -> w276
          frame "av2" {
            n103 = property on="Set switches 2" class="Arr (strict)"(error in=w286) -> (error out=w285:errorcluster, "Value"=w287:bool[])  [unwired: 1 in, 1 out]
          }
          frame Default {
          }
          frame "av1" {
            n104 = property on="Set switches" class="Arr (strict)"(error in=w292) -> (error out=w291:errorcluster, "Value"=w293:bool[])  [unwired: 1 in, 1 out]
          }
        }
        n105 = Unbundle By Name(w278) -> ("Toggle On/Off"=w274:bool)
        n106 = call "Avocent_build_command_toggle.vi"("Set switches"=w273, "Toggle On/Off"=w274) -> ("HTTP Command"=w275:string)  [unwired: 9 in]
        n107 = Bundle By Name(cluster=w278, "HTTP Command"=w275) -> (w282:T3)
        n108 = call <vilib>:"Add State(s) to Queue__jki_lib_state_machine.vi"("State(s) in (\"\")"=w276) -> ("States Out"=w283:string)  [unwired: 14 in]
      }
      frame "action:update status" {
        # "Your code here.\n(You can make a copy of, or modify, this frame)"
        n109 = Unbundle By Name(w301) -> ("Power Status"=w294:string)
        n110 = call "Avocent_power_status.vi"("Power Status (raw string)"=w294) -> ("Power status (boolean)"=w295:bool[])  [unwired: 10 in]
        n111 = case shown="\"av2\"" w300 {
          tunnel: w295 -> [w305 _ w310]
          tunnel: w299 -> [w304 _ w309]
          tunnel: [w304 errorcluster {"status"=TRUE, "code"=0, "source"="Error:\nno avocent selected"} ("error out") w309] -> w298
          tunnel: w297 -> [w303 _ w308]
          tunnel: [w303 "" w308] -> w296
          frame "av2" {
            "Power indicator 2" <- w305
          }
          frame Default {
          }
          frame "av1" {
            "Power indicator" <- w310
          }
        }
        n112 = call <vilib>:"Add State(s) to Queue__jki_lib_state_machine.vi"("State(s) in (\"\")"=w296) -> ("States Out"=w302:string)  [unwired: 14 in]
      }
      frame "action:get status cmd" {
        # "Your code here.\n(You can make a copy of, or modify, this frame)"
        n113 = Bundle By Name(cluster=w313, "HTTP Command"="/control.cgi" ("Command")) -> (w312:T3)
        n114 = call <vilib>:"Add State(s) to Queue__jki_lib_state_machine.vi"("State(s) in (\"\")"=w316) -> ("States Out"=w315:string)  [unwired: 14 in]
      }
      frame "action:set to current values" {
        # "Your code here.\n(You can make a copy of, or modify, this frame)"
        n115 = property on="Power indicator" class="Arr (strict)"(error in=w319) -> (error out=w320:errorcluster, "Value"=w317:bool[])  [unwired: 1 in, 1 out]
        n116 = property on="Set switches" class="Arr (strict)"(error in=w320, "Val(Sgnl)"=w317) -> (error out=w318:errorcluster)  [unwired: 1 in, 1 out]
        n117 = call <vilib>:"Add State(s) to Queue__jki_lib_state_machine.vi"("State(s) in (\"\")"=w323) -> ("States Out"=w322:string)  [unwired: 14 in]
      }
      frame "action:set to current values 2" {
        # "Your code here.\n(You can make a copy of, or modify, this frame)"
        n118 = property on="Power indicator 2" class="Arr (strict)"(error in=w327) -> (error out=w325:errorcluster, "Value"=w324:bool[])  [unwired: 1 in, 1 out]
        n119 = property on="Set switches 2" class="Arr (strict)"(error in=w325, "Val(Sgnl)"=w324) -> (error out=w326:errorcluster)  [unwired: 1 in, 1 out]
        n120 = call <vilib>:"Add State(s) to Queue__jki_lib_state_machine.vi"("State(s) in (\"\")"=w330) -> ("States Out"=w329:string)  [unwired: 14 in]
      }
      frame "action: set to all on/off" {
        # "Your code here.\n(You can make a copy of, or modify, this frame)"
        n121 = Unbundle By Name(w332) -> ("Set all On/Off"=w334:bool)
        n122 = Initialize Array(w334, 16 ("dimension size")) -> (w331:bool[])
        n123 = case shown="\"av2\"" w337 {
          tunnel: w339 -> [w343 _ w349]
          tunnel: [w342 errorcluster {"status"=TRUE, "code"=0, "source"="Error:\nno avocent selected"} ("error out") w348] -> w338
          tunnel: w336 -> [w344 _ w350]
          tunnel: [w344 "" w350] -> w335
          tunnel: w331 -> [w341 _ w347]
          frame "av2" {
            n124 = property on="Set switches 2" class="Arr (strict)"(error in=w343, "Val(Sgnl)"=w341) -> (error out=w342:errorcluster)  [unwired: 1 in, 1 out]
          }
          frame Default {
          }
          frame "av1" {
            n125 = property on="Set switches" class="Arr (strict)"(error in=w349, "Val(Sgnl)"=w347) -> (error out=w348:errorcluster)  [unwired: 1 in, 1 out]
          }
        }
        n126 = call <vilib>:"Add State(s) to Queue__jki_lib_state_machine.vi"("State(s) in (\"\")"=w335) -> ("States Out"=w340:string)  [unwired: 14 in]
      }
      frame "action: update labels" {
        n127 = call "get software root directory.vi"() -> ("Application Directory"=w361:path)  [unwired: 11 in]
        n128 = Strip Path(path=w361) -> (stripped path=w360:path)  [unwired: 1 out]
        n129 = Build Path(base path=w360, name or relative path="user data\\Avocent_PSU_Labels.txt") -> (appended path=w359:path)
        n130 = call <vilib>:"Open Config Data.vi"("error in (no error)"=w356, "create file if necessary (T)"=FALSE, "configuration file path"=w359) -> ("error out"=w357:errorcluster, "refnum"=w358:T5)  [unwired: 6 in, 1 out]
        n131 = case shown="\"av1\"" w351 {
          selector: w351 -> [_ _ w368]
          tunnel: ["Avocent-PSU-upstream" ("section") "Avocent-PSU-downstream" ("section") w369] -> w352
          frame "av1" {
          }
          frame "av2" {
          }
          frame Default {
            n132 = String Subset(string=w368, offset (0)=2) -> (substring=w370:string)  [unwired: 1 in]
            n133 = Concatenate Strings("Avocent " ("section"), w370) -> (w369:string)
          }
        }
        n134 = for {
          N: 16 -> [_]
          tunnel: w358 -> [w385]
          tunnel: w357 -> [w384]
          tunnel: [w383] -> w355
          tunnel: [w382] -> w354 mode=indexing
          tunnel: w352 -> [w375]
          i -> [w377]
          n135 = Add(x=w377, y=1) -> (x+y=w378:i32)
          n136 = Number To Decimal String(number=w378) -> (decimal integer string=w380:string)  [unwired: 1 in]
          n137 = Concatenate Strings("Label " ("key"), w380) -> (w379:string)
          n138 = call-poly <vilib>:"Read Key.vi"("section"=w375, "error in (no error)"=w384, "default value"="", "key"=w379, "refnum"=w385) -> ("error out"=w383:errorcluster, "value"=w382:string)  [unwired: 3 in, 2 out]
        }
        n139 = case shown="\"av1\"" w351 {
          tunnel: w354 -> [w373 w374 _]
          frame "av1" {
            "Avocent Labels Av1" <- w373
          }
          frame "av2" {
            "Avocent Labels Av2" <- w374
          }
          frame Default {
          }
        }
      }
    }
  }
